vi "Main Control Globals.vi"() -> ()   [LabVIEW 2021]
panel:
  out "Exit":bool
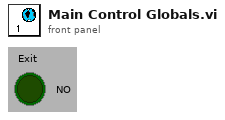
[diagram p1: front panel]
diagram:
